vi "Read Container.vi"(6 "Queue timeout in ms (-1)":i32=-1, 8 "error in (no error)":errorcluster, 9 "Read from SHV (F)":bool, 11 "Transfer Line in":refnum<class "Transfer Line.lvclass">) -> (0 "error out":errorcluster, 1 "Sample":refnum<class "Sample.lvclass">, 2 "Sample Container":T1, 3 "Transfer Line out":refnum<class "Transfer Line.lvclass">, 4 "Overflow Sample":refnum<class "Sample.lvclass">)   [LabVIEW 2015, in "cRIO-Carbondioxide.lvlib" / "CO2-Actor.lvlib" / "Transfer Line.lvclass"]
uses:
  Transfer Line.lvclass
  Controls/Sample Container.ctl
  subs/Sample/Sample.lvclass
  Transfer Line.lvclass/Transfer Line.ctl
panel:
  out "Queue timed out?":bool
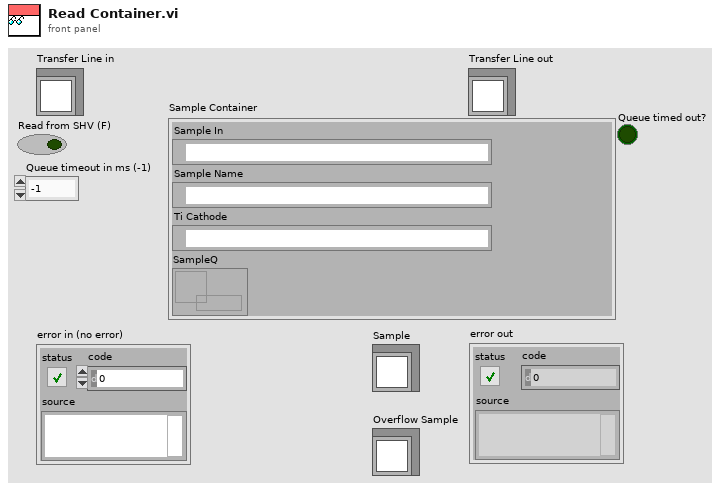
[diagram p1: front panel]
types:
  T1 = typedef "Sample Container.ctl" = cluster{"Sample In":refnum<k21>, "Sample Name":refnum<k21>, "Ti Cathode":refnum<k21>, "SampleQ":refnum<queue>}
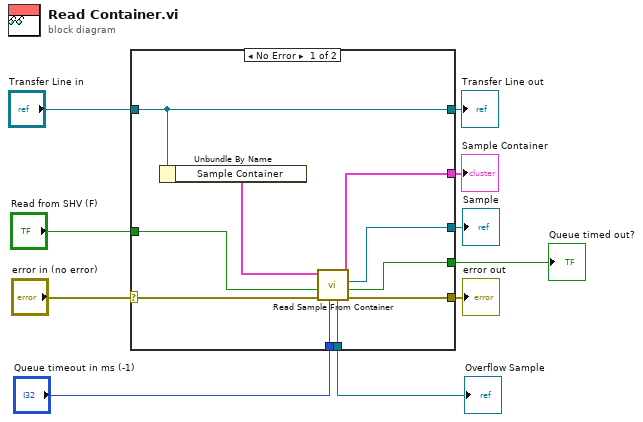
[diagram p0: block diagram]
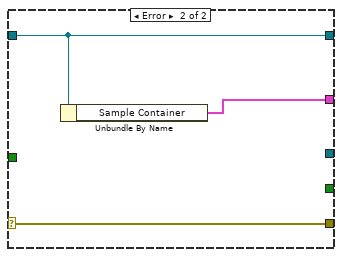
[diagram p2: hidden frame]
diagram:
  n1 = case shown="No Error" "error in (no error)" {
    selector: "error in (no error)" -> [w19 w23]
    tunnel: [w18 w23] -> w9
    tunnel: [w14 _] -> w8
    tunnel: "Transfer Line in" -> [w20 w22]
    tunnel: [w20 w22] -> w6
    tunnel: [w16 w21] -> w5
    tunnel: "Read from SHV (F)" -> [w15 _]
    tunnel: "Queue timeout in ms (-1)" -> [w13 _]
    tunnel: [w12 _] -> w2
    tunnel: [w11 _] -> w1
    frame No Error {
      n2 = Unbundle By Name(w20) -> ("Sample Container"=w17:T1)
      n3 = call "Read Sample From Container.vi"("Queue timeout in ms (-1)"=w13, "error in (no error)"=w19, "Read from SHV (F)"=w15, "Container"=w17) -> ("error out"=w18:errorcluster, "Queue timed out?"=w11:bool, "Sample out"=w14:refnum<class "Sample.lvclass">, "Container"=w16:T1, "Overflow Sample"=w12:refnum<class "Sample.lvclass">)  [unwired: 3 in]
    }
    frame Error {
      n4 = Unbundle By Name(w22) -> ("Sample Container"=w21:T1)
    }
  }
  "Transfer Line out" <- w6
  "Sample Container" <- w5
  "error out" <- w9
  "Sample" <- w8
  "Overflow Sample" <- w2
  "Queue timed out?" <- w1
